vi "Cash.vi"(8 "error in (no error)":errorcluster, 10 "Cash":T1, 11 "Actor_USD in":refnum<class "Actor_USD.lvclass">) -> (0 "error out":errorcluster, 3 "Actor_USD out":refnum<class "Actor_USD.lvclass">)   [LabVIEW 2019, in "Actor_USD.lvlib" / "Actor_USD.lvclass"]
uses:
  Actor_USD.lvclass
  C:/Program Files/National Instruments/LabVIEW 2019/vi.lib/ActorFramework/Actor/Actor.lvclass
  <vilib>/ActorFramework/Actor/Actor.lvclass/Actor.ctl
  Actor_USD.lvclass/Actor_USD.ctl
  UI Actor Messages/Update Credit Msg/Update Credit Msg.lvclass/Update Credit Msg.ctl
  <vilib>/ActorFramework/Message Enqueuer/Message Enqueuer.lvclass/Message Enqueuer.ctl
  <vilib>/ActorFramework/Message Enqueuer/Enqueue.vi
  UI Actor Messages/Update Credit Msg/Update Credit Msg.lvclass
  C:/Program Files/National Instruments/LabVIEW 2019/vi.lib/ActorFramework/Message/Message.lvclass
  <vilib>/ActorFramework/Message Priority Queue/Priority Enqueue.vi
  <vilib>/ActorFramework/Actor/Actor.lvclass
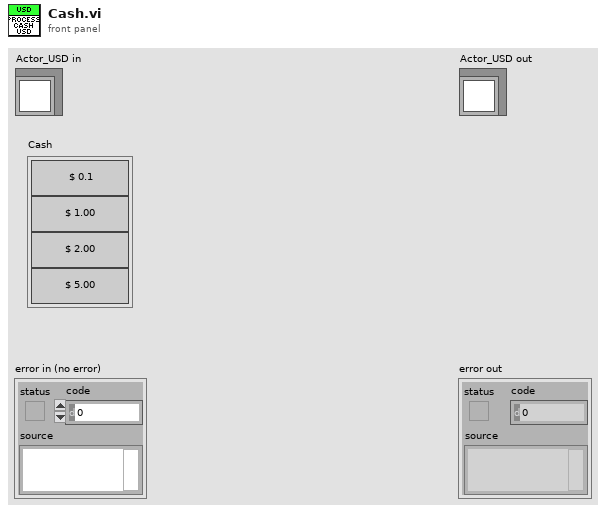
[diagram p1: front panel]
types:
  T1 = cluster{"1 P":bool, "2 P":bool, "5P":bool, "10 P":bool}
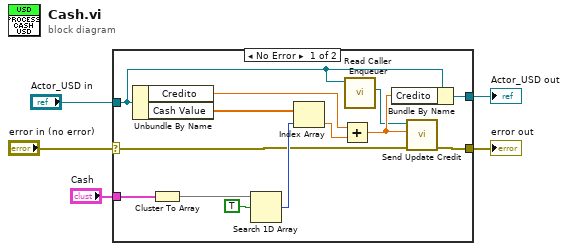
[diagram p0: block diagram]
diagram:
  n1 = case shown="No Error" "error in (no error)" {
    selector: "error in (no error)" -> [w9 w20]
    tunnel: [w8 w20] -> w4
    tunnel: [w11 w19] -> w2
    tunnel: "Actor_USD in" -> [w7 w19]
    tunnel: "Cash" -> [w18 _]
    frame No Error {
      n2 = Unbundle By Name(w7) -> ("Credito"=w13:dbl, "Cash Value"=w14:dbl[])
      n3 = Cluster To Array(cluster=w18) -> (array=w17:bool[])
      n4 = Search 1D Array(1D array=w17, element=TRUE) -> (index of element=w15:i32)  [unwired: 1 in]
      n5 = Index Array(array=w14, index=w15) -> (element=w12:dbl)
      n6 = Add(x=w13, y=w12) -> (x+y=w10:dbl)
      n7 = call <vilib>:"Read Caller Enqueuer.vi"("Actor"=w7) -> ("Caller Enqueuer"=w6:refnum<class "Message Enqueuer.lvclass">)  [unwired: 10 in]
      n8 = Bundle By Name(cluster=w7, "Credito"=w10) -> (w11:refnum<class "Actor_USD.lvclass">)
      n9 = call "Send Update Credit.vi"("error in (no error)"=w9, "Credito"=w10, "Message Enqueuer"=w6) -> ("error out"=w8:errorcluster)  [unwired: 7 in, 1 out]
    }
    frame Error {
    }
  }
  "error out" <- w4
  "Actor_USD out" <- w2
